vi "SiCM.vi"() -> ()   [LabVIEW 2016]
doc: "SICM module for Hopping Mode.\nRunning this VI takes the control over the PID (ZController). But closing it by clicking on the Cross in the corner of the window releases the PID which is accessible again.\nTo use the motor and the auto-approach module, the window ZController should be used while the SICM Hopping window is running. The Z Controller window will do the Auto-Approach by turning on and off the Hopping movement."
uses:
  controls/Enum.ctl
  <vilib>/rvi/interface/common/niFpgaWaitOnOcc.vi
  <vilib>/rvi/errors/niLvFpgaAdjustHostInterfaceError.vi
  <vilib>/RVI Host/nirviSupport.llb/nirviErrorClusterFromErrorCode.vi
  <vilib>/rvi/interface/nirviMethod/nirviMethod.xnode
  controls/FPGAVIreferenceTypeDef.ctl
  FPGA Bitfiles/qnmController797_usbRIO_controllerFPGAmu.lvbitx
  <vilib>/rvi/interface/nirviReadWriteControl/nirviReadWriteControl.xnode
  <vilib>/regexp/Match Regular Expression.xnode
  controls/FPGAVIreferenceTypeDefScanEngine.ctl
  Course Project/support/Message Queue/Message Queue.lvlib
  <vilib>/rvi/errors/niLvFpgaMergeErrorWithErrorCode.vi
  Course Project/support/User Event - Stop/User Event - Stop.lvlib
  <vilib>/FPGAPlugInAG/USB-7856R OEM/niLvFpga_AcknowledgeIrq_USB-7856R OEM.vi
  NiFpgaLv.dll
  <vilib>/FPGAPlugInAG/USB-7856R OEM/niLvFpga_ReadFifo_USB-7856R OEM.vi
  <vilib>/FPGAPlugInAG/USB-7856R OEM/niLvFpga_ConfigureFifo_USB-7856R OEM.vi
  <vilib>/FPGAPlugInAG/USB-7856R OEM/niLvFpga_StartFifo_USB-7856R OEM.vi
  <vilib>/rvi/interface/nirviMethod/StockFPGA_InlinedMethodWaitForSingleIRQ.vi
  <vilib>/FPGAPlugInAG/USB-7856R OEM/niLvFpga_WaitOnIrq_USB-7856R OEM.vi
  <vilib>/FPGAPlugInAG/USB-7856R OEM/niLvFpga_StopFifo_USB-7856R OEM.vi
panel:
  out "Progress":u8(slide) scale=0.0..100.0
  out "Cursor":dbl format="%#_3pm"
  out "Trig Height":dbl=1.0953788757324218e-07 format="%#_3pm"
  in  "Plots":T1={"Current"=TRUE, "Baseline"=TRUE, "Height"=TRUE, "TrigHeight"=TRUE}
  in  "Real Time":bool
  in  "Update":i32=20 format="%.0fms"
  in  "Window":cluster{"Window":dbl}={"Window"=0.005} {"Window" format="%_3ps"}
  out "Baseline":dbl=0.9660243988037109 format="%#_3p"
  out "Height":dbl=-5.129915237426758e-07 format="%#_3pm"
  out "Current":dbl=0.96649169921875 format="%#_3p"
  in  "SICM":enum32{"Hopping", "IV Curve"}(tab)
  in  "Retract period":dbl=0.002048131080389145 format="%#_3ps"
  in  "Enable?":bool caption="Enable"
  in  "Setpoint":sgl=99.0 min=0 max=100 format="%_3g%"
  in  "Retract height":dbl=2e-06 min=0.0 max=5e-06 format="%_3pm"
  in  "Approach rate":dbl=0.0001 format="%_3pm/s"
  in  "Adaptive":bool=TRUE
  in  "Retract delay":dbl=0.0009379999999999996 min=1e-09 format="%_3ps"
  in  "Adaptive min":dbl=9.0 format="%#_3f%"
  in  "Average period":dbl=0.001 min=1e-09 format="%_3ps"
  in  "Time constant":dbl=3.0 min=1e-09 format="%#_3ps"
  in  "Delta":dbl=5.55e-05 format="%_3p"
  in  "Relative":bool=TRUE
  in  "Ramp":bool caption="Enable"
  out "Inner radius":dbl format="%#_3pm"
  out "Resistance":dbl format="%#_3pOhm"
  out "Z":dbl=0.1 format="%.0pV"
  out "XY":dbl=0.1 format="%.0pV"
  out "R²":dbl=0.1 format="%_3f%"
  in  "IVParameters":T2={"Solution"="140", "Gain"=1.0, "Conductivity"=140.0, "Apex Angle"=5.0, "Points"=100, "Voltage\nRamp"={"Min"=-3.0, "Max"=3.0}} {"Voltage\nRamp"."Min" format="%#_3pV"; "Voltage\nRamp"."Max" format="%#_3pV"; "Points" format="%#.0f"; "Apex Angle" format="%#_3pdeg"; "Conductivity" format="%#_3pS/m"; "Gain" format="%#_3p"}
  out "IV Curve":cluster{dbl[], dbl[]}(graph)
  in  "Reset":bool
  out "Graph":waveform(dbl)[](graph)
  out "RT Graph":dbl[][](graph)
  # "Baseline"
  # "Hopping"
  # "Baseline"
  # "Resolution"
  # "Display"
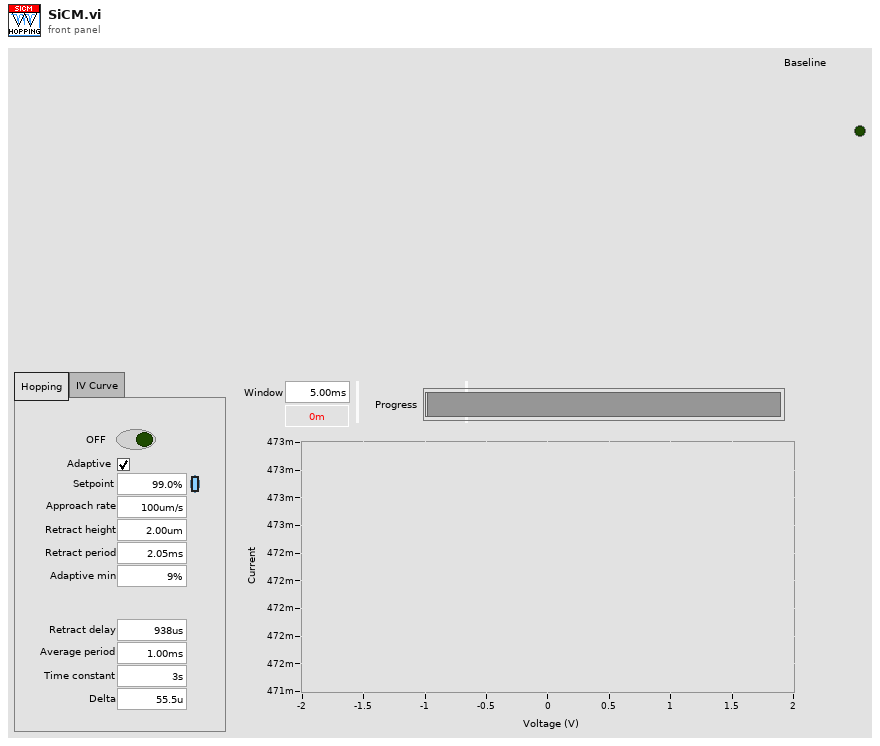
[diagram p1: front panel]
types:
  T1 = cluster{"Current":bool, "Baseline":bool, "Height":bool, "TrigHeight":bool}
  T2 = cluster{"Solution":string, "Gain":dbl, "Conductivity":dbl, "Apex Angle":dbl, "Points":i32, "Voltage\nRamp":cluster{"Min":dbl, "Max":dbl}}
  T3 = typedef "Enum.ctl" = enum16{"Init", "Read", "Write"}
  T4 = cluster{"calibName":string[], "calibParameters":cluster{"Sensitivity":cluster{"Sens X":dbl, "Sens Y":dbl, "Sens Z":dbl}, "Range":cluster{"Range X":dbl, "Range Y":dbl, "Range Z":dbl}, "HV gain":cluster{"HV gain X":dbl, "HV gain Y":dbl, "HV gain Z":dbl}}[], "calibIndex":i32}
  T5 = cluster{"Sensitivity":cluster{"Sens X":dbl, "Sens Y":dbl, "Sens Z":dbl}, "Range":cluster{"Range X":dbl, "Range Y":dbl, "Range Z":dbl}, "HV gain":cluster{"HV gain X":dbl, "HV gain Y":dbl, "HV gain Z":dbl}}[]
  T6 = typedef "FPGAVIreferenceTypeDef.ctl" = refnum<k20>
  T7 = cluster{"Sensitivity":cluster{"Sens X":dbl, "Sens Y":dbl, "Sens Z":dbl}, "Range":cluster{"Range X":dbl, "Range Y":dbl, "Range Z":dbl}, "HV gain":cluster{"HV gain X":dbl, "HV gain Y":dbl, "HV gain Z":dbl}}
  T8 = typedef "Message Queue.lvlib/All Message Queues.ctl" = cluster{"IU":refnum<queue>}
  T9 = typedef "FPGAVIreferenceTypeDefScanEngine.ctl" = refnum<k20>
  T10 = cluster{"write":bool, "data":fxp<+,16,1>, "index":u16}
  T11 = enum8{"Enabled", "Disabled", "Disabled and Grayed Out"}
  T12 = cluster{"inverseDecimation":fxp<+,22,0>, "decimation":u16, "waveSize":u16, "pixelDecimation":u16}
  T13 = cluster{"sicm.p.enable":bool, "sicm.p.adaptiveStepDown":bool, "sicm.p.relSetpoint":bool}
  T14 = cluster{"sicm.p.setPoint":fxp<+,20,0>, "sicm.p.setPointFrac":fxp<+/-,20,14>, "stepDown":fxp<+/-,28,4>, "retractHeight":fxp<+/-,28,4>, "adaptiveMin":fxp<+,10,0>}
  T15 = cluster{"scanEngineHz":u32, "feedbackHz":u32, "sicmHz":u32, "rampHz":u32}
  T16 = cluster{"se.blc.p.postRetractDelay":u16, "se.blc.p.windowSize":u16, "se.blc.p.updateFactor":i16, "blc.resetBackground":bool, "se.blc.p.mindelta":fxp<+/-,12,-14>}
  T17 = cluster{"hdt.int.s.transferSource":u8, "hdt.int.p.useInternalMemStartPos":bool, "hdt.int.p.memStartPos":fxp<+,14,14>, "hdt.int.p.readLength":u16, "hdt.int.p.readFwd":bool, "hdt.int.p.memReadDec":u16, "hdt.int.p.startTransfer":bool}
  T18 = cluster{"sicm.ptsAfterTrig":u16, "sicm.p.memorywWriteDec":u16}
  T19 = cluster{"feedbackHz":u32, "sicm.display.sicm.p.memorywWriteDec":u16}
  T20 = cluster{"carryOut":fxp<+/-,22,2>, "1/x":fxp<+/-,32,24>, "x*y":fxp<+,24,1>}
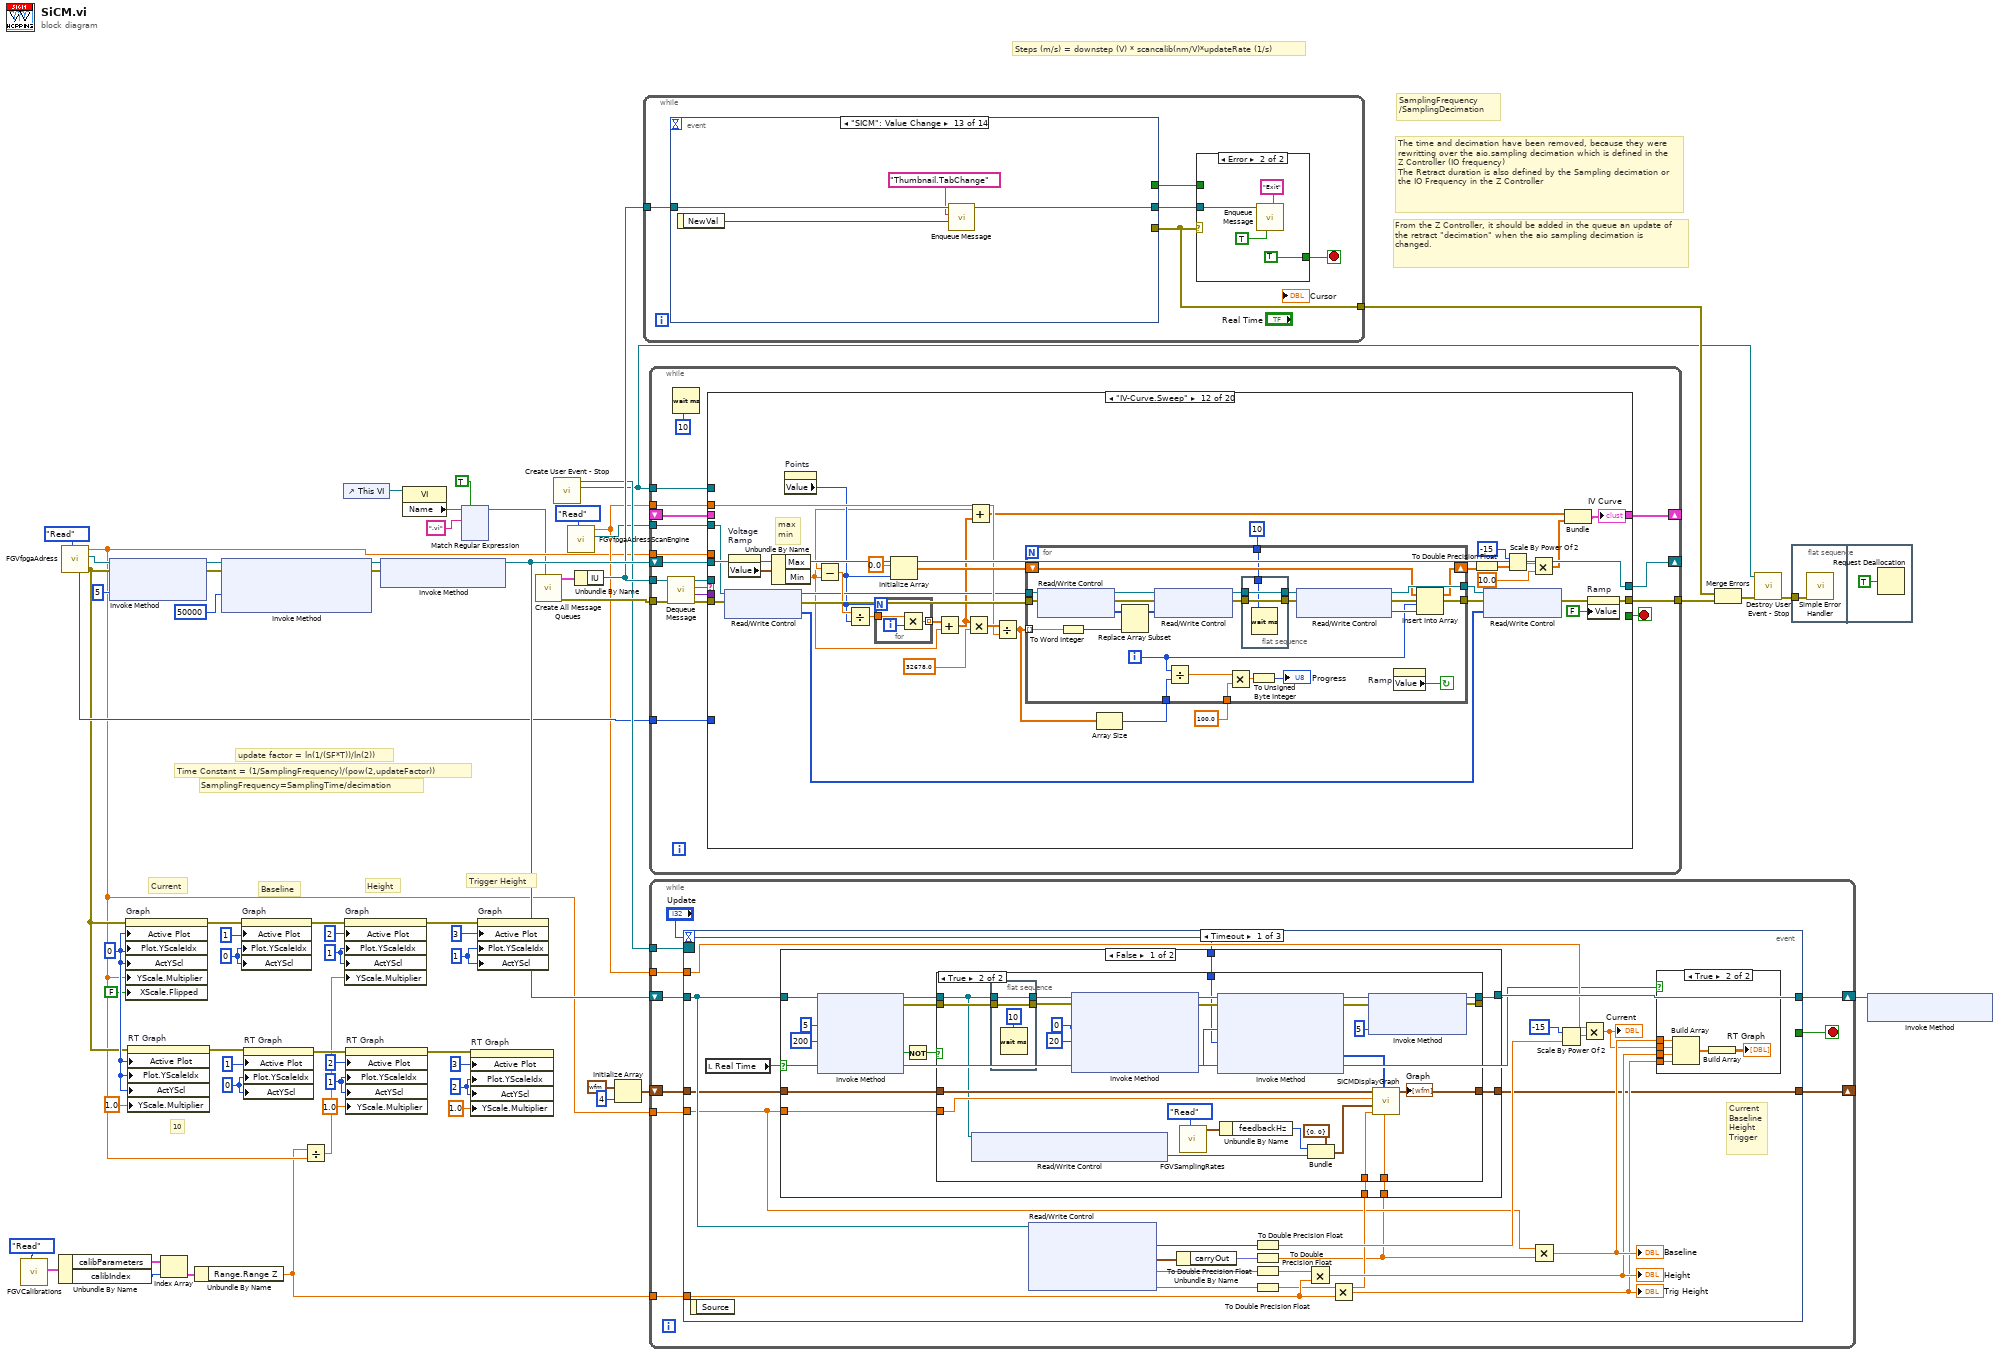
[diagram p0: block diagram]
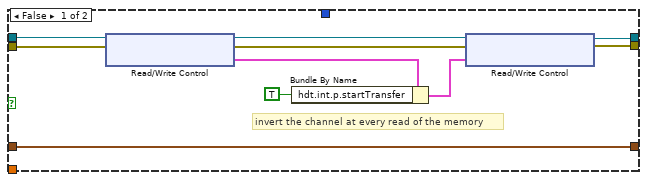
[diagram p2: hidden frame]
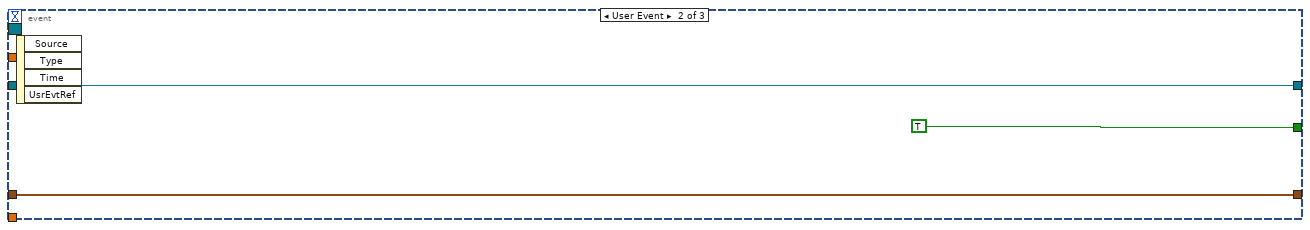
[diagram p5: hidden frame]
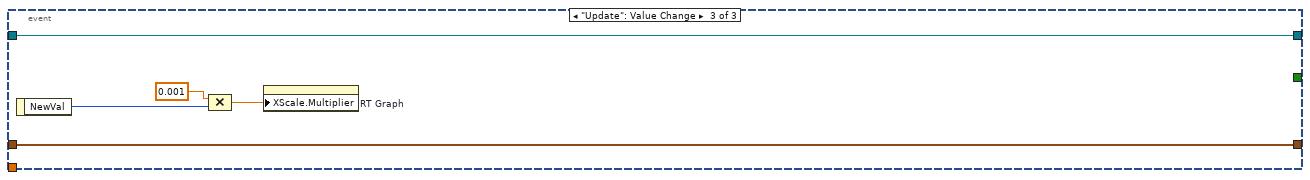
[diagram p6: hidden frame]
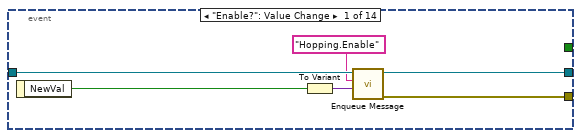
[diagram p8: hidden frame]
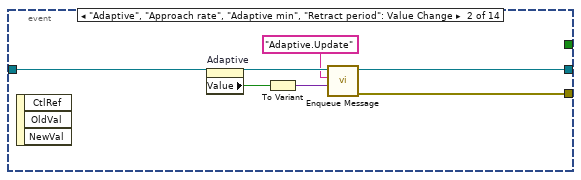
[diagram p9: hidden frame]
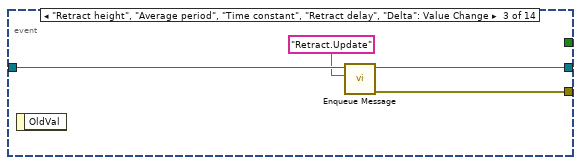
[diagram p10: hidden frame]
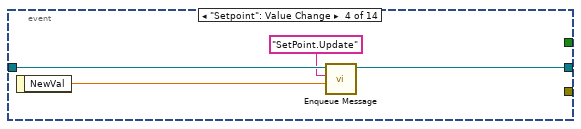
[diagram p11: hidden frame]
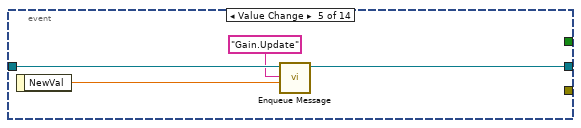
[diagram p12: hidden frame]
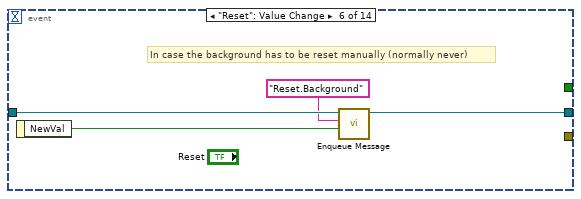
[diagram p13: hidden frame]
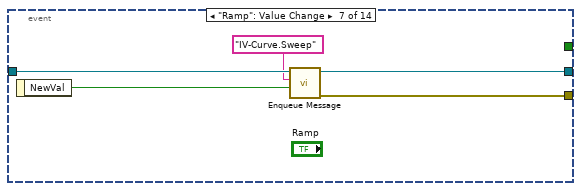
[diagram p14: hidden frame]
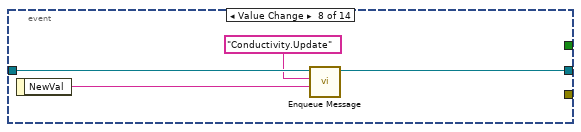
[diagram p15: hidden frame]
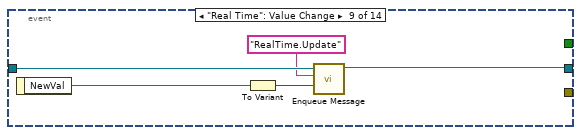
[diagram p16: hidden frame]
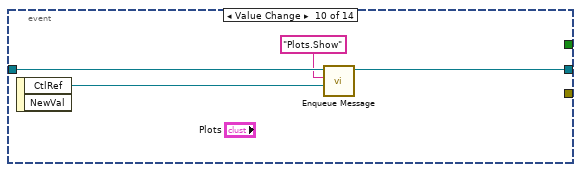
[diagram p17: hidden frame]
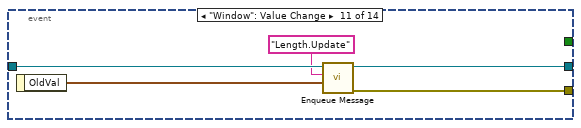
[diagram p18: hidden frame]
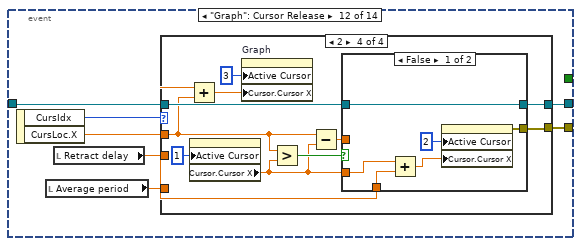
[diagram p19: hidden frame]
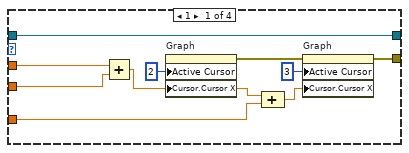
[diagram p20: hidden frame]
diagram:
  w20 = 2 ("Active Y Scale")
  w23 = 1 ("Active Y Scale")
  w26 = 0 ("Active Y Scale")
  w31 = 1 ("Active Y Scale")
  w33 = 1 ("Active Y Scale")
  w27 = u32 0 ("Active Plot")
  w35 = 0 ("Active Y Scale")
  # "10"
  # "Baseline"
  # "Current"
  # "Trigger Height"
  # "Height"
  # "From the Z Controller, it should be added in the queue an update of the retract \"decimation\" when the aio sampling decimation is changed."
  # "The time and decimation have been removed, because they were rewritting over the aio.sampling decimation which is defined in the Z Controller (IO frequency)\nThe Retract duration is also defined by the Sampling decimation or the IO Frequency in the Z Controller"
  # "SamplingFrequency\n/SamplingDecimation"
  # "SamplingFrequency=SamplingTime/decimation"
  # "update factor = ln(1/(SF*T))/ln(2))"
  # "Time Constant = (1/SamplingFrequency)/(pow(2,updateFactor))"
  # "Steps (m/s) = downstep (V) * scancalib(nm/V)*updateRate (1/s)"
  n1 = call "FGVCalibrations.vi"("Enum"=Enum."Read") -> ("calibOut"=w38:T4)  [unwired: 9 in, 1 out]
  n2 = Unbundle By Name(w38) -> ("calibParameters"=w39:T5, "calibIndex"=w41:i32)
  n3 = call "FGVfpgaAdress.vi"("Enum"=Enum."Read") -> ("error out"=w17:errorcluster, "FPGA VI Reference Out"=w61:T6, "voltageRange(+/-)Out"=w14:dbl, "ioFreqHzOut"=w44:u32)  [unwired: 5 in, 2 out]
  n4 = xnode "Invoke Method"("FPGA VI Reference In"=w61, "error in"=w17, "IRQ Number(s)"=5) -> ("FPGA VI Reference Out"=w50:T6, "error out"=w51:errorcluster)
  n5 = property on="Graph" class="WFGraph (strict)"(error in=w17, "Active Plot"=w27, "Plot.YScaleIdx"=w27, "ActYScl"=w27, "YScale.Multiplier"=w14, "XScale.Flipped"=FALSE ("X Scale.Flipped")) -> (error out=w30:errorcluster)  [unwired: 1 in, 1 out]
  n6 = property on="RT Graph" class="WFChart (strict)"(error in=w17, "Active Plot"=w27, "Plot.YScaleIdx"=w27, "ActYScl"=w27, "YScale.Multiplier"=1.0 ("Y Scale.Offset and Multiplier:Multiplier")) -> (error out=w24:errorcluster)  [unwired: 1 in, 1 out]
  n7 = Index Array(array=w39, index=w41) -> (element=w40:T7)
  n8 = Unbundle By Name(w40) -> ("Range.Range Z"=w11:dbl)
  n9 = xnode "Invoke Method"("FPGA VI Reference In"=w50, "error in"=w51, "Requested Depth"=u32 50000) -> ("FPGA VI Reference Out"=w55:T6, "error out"=w53:errorcluster)  [unwired: 1 out]
  n10 = property on="Graph" class="WFGraph (strict)"(error in=w30, "Active Plot"=u32 1, "Plot.YScaleIdx"=w35, "ActYScl"=w35) -> (error out=w29:errorcluster)  [unwired: 1 in, 1 out]
  n11 = property on="RT Graph" class="WFChart (strict)"(error in=w24, "Active Plot"=u32 1, "Plot.YScaleIdx"=w26, "ActYScl"=w26) -> (error out=w21:errorcluster)  [unwired: 1 in, 1 out]
  n12 = Divide(x=w11, y=w14) -> (x/y=w13:dbl)
  n13 = control-ref of="This VI"() -> (w5:refnum<vi>)
  n14 = property on="Graph" class="WFGraph (strict)"(error in=w29, "Active Plot"=u32 2, "Plot.YScaleIdx"=w33, "ActYScl"=w33, "YScale.Multiplier"=w13) -> (error out=w28:errorcluster)  [unwired: 1 in, 1 out]
  n15 = property on="RT Graph" class="WFChart (strict)"(error in=w21, "Active Plot"=u32 2, "Plot.YScaleIdx"=w23, "ActYScl"=w23, "YScale.Multiplier"=1.0 ("Y Scale.Offset and Multiplier:Multiplier")) -> (error out=w18:errorcluster)  [unwired: 1 in, 1 out]
  n16 = xnode "Invoke Method"("FPGA VI Reference In"=w55, "error in"=w53) -> ("FPGA VI Reference Out"=w63:T6)  [unwired: 1 out]
  n17 = property class="VI"(reference=w5) -> ("Name"=w4:string)  [unwired: 1 in, 2 out]
  n18 = xnode "Match Regular Expression"("input string"=w4, "regular expression"=".vi", "ignore case? (F)"=TRUE) -> ("before match"=w2:string)  [unwired: 3 in, 4 out]
  n19 = property on="RT Graph" class="WFChart (strict)"(error in=w18, "Active Plot"=u32 3, "Plot.YScaleIdx"=w20, "ActYScl"=w20, "YScale.Multiplier"=1.0 ("Y Scale.Offset and Multiplier:Multiplier")) -> ()  [unwired: 1 in, 2 out]
  n20 = property on="Graph" class="WFGraph (strict)"(error in=w28, "Active Plot"=u32 3, "Plot.YScaleIdx"=w31, "ActYScl"=w31) -> ()  [unwired: 1 in, 2 out]
  n21 = call "Create All Message Queues.vi"("QueueName"=w2) -> ("ErrorOut"=w58:errorcluster, "MessageQueueOut"=w60:T8)  [unwired: 9 in]
  n22 = call "Create User Event - Stop.vi"() -> ("Événement utilisateur - Arrêt"=w46:refnum<user-event>, "Refnum Enregistrement à l'événement Arrêt"=w49:refnum<event-registration>)  [unwired: 9 in, 1 out]
  n23 = call "FGVfpgaAdressScanEngine.vi"("Enum"=Enum."Read") -> ("FPGA.SEout"=w45:T9, "voltageRange(+/-)Out"=w42:dbl)  [unwired: 6 in, 3 out]
  n24 = Unbundle By Name(w60) -> ("IU"=w59:refnum<queue>)
  n25 = Initialize Array(waveform(dbl) {"t0"=timestamp(0 s since 1904-01-01), "dt"=1.0, "Y"=[0.0]}, 4 ("dimension size")) -> (w8:waveform(dbl)[])
  n26 = while {
    tunnel: w59 -> [w68]
    tunnel: [w64] -> w56
    stop <- w66 stop-if-true
    n27 = event shown="[12] \"SICM\": Value Change" {
      selector: _ -> [_ _ _ _ _ _ _ _ _ _ _ _ _ _]
      dyn-events: _ -> [_ _ _ _ _ _ _ _ _ _ _ _ _ _]
      timeout: _ -> [_ _ _ _ _ _ _ _ _ _ _ _ _ _]
      tunnel: [_ _ _ _ _ _ _ _ _ _ _ _ _ w197] -> w67
      tunnel: w68 -> [w79 w85 w89 w93 w97 w101 w106 w110 w115 w119 w124 w131 w191 w193]
      tunnel: [w76 w82 w86 _ _ _ w103 _ _ _ w121 w127 _ _] -> w64
      tunnel: [w78 w83 w87 w91 w96 w100 w104 w109 w114 w118 w122 w130 w190 w192] -> w65
      event "Enable?": Value Change {
        n28 = event-data() -> ("NewVal"=w75:bool)  [unwired: 1 in]
        n29 = To Variant(anything=w75) -> (Variant=w74:variant)
        n30 = call "Enqueue Message.vi"("Data"=w74, "Message"="Hopping.Enable", "Queue"=w79) -> ("error out"=w76:errorcluster, "Queue dup."=w78:refnum<queue>)  [unwired: 7 in]
      }
      event "Adaptive", "Approach rate", "Adaptive min", "Retract period": Value Change {
        n31 = event-data() -> ()  [unwired: 1 in, 3 out]
        n32 = property on="Adaptive" class="Bool (strict)"() -> ("Value"=w81:bool)  [unwired: 2 in, 2 out]
        n33 = To Variant(anything=w81) -> (Variant=w80:variant)
        n34 = call "Enqueue Message.vi"("Data"=w80, "Message"="Adaptive.Update", "Queue"=w85) -> ("error out"=w82:errorcluster, "Queue dup."=w83:refnum<queue>)  [unwired: 7 in]
      }
      event "Retract height", "Average period", "Time constant", "Retract delay", "Delta": Value Change {
        n35 = event-data() -> ()  [unwired: 1 in, 1 out]
        n36 = call "Enqueue Message.vi"("Message"="Retract.Update", "Queue"=w89) -> ("error out"=w86:errorcluster, "Queue dup."=w87:refnum<queue>)  [unwired: 8 in]
      }
      event "Setpoint": Value Change {
        n37 = event-data() -> ("NewVal"=w90:sgl)  [unwired: 1 in]
        n38 = call "Enqueue Message.vi"("Data"=w90, "Message"="SetPoint.Update", "Queue"=w93) -> ("Queue dup."=w91:refnum<queue>)  [unwired: 7 in, 1 out]
      }
      event "IVParameters.Gain": Value Change {
        n39 = event-data() -> ("NewVal"=w94:dbl)  [unwired: 1 in]
        n40 = call "Enqueue Message.vi"("Data"=w94, "Message"="Gain.Update", "Queue"=w97) -> ("Queue dup."=w96:refnum<queue>)  [unwired: 7 in, 1 out]
      }
      event "Reset": Value Change {
        # "In case the background has to be reset manually (normally never)"
        n41 = event-data() -> ("NewVal"=w98:bool)  [unwired: 1 in]
        n42 = call "Enqueue Message.vi"("Data"=w98, "Message"="Reset.Background", "Queue"=w101) -> ("Queue dup."=w100:refnum<queue>)  [unwired: 7 in, 1 out]
      }
      event "Ramp": Value Change {
        n43 = event-data() -> ("NewVal"=w102:bool)  [unwired: 1 in]
        n44 = call "Enqueue Message.vi"("Data"=w102, "Message"="IV-Curve.Sweep", "Queue"=w106) -> ("error out"=w103:errorcluster, "Queue dup."=w104:refnum<queue>)  [unwired: 7 in]
      }
      event "IVParameters.Solution": Value Change {
        n45 = event-data() -> ("NewVal"=w107:string)  [unwired: 1 in]
        n46 = call "Enqueue Message.vi"("Data"=w107, "Message"="Conductivity.Update", "Queue"=w110) -> ("Queue dup."=w109:refnum<queue>)  [unwired: 7 in, 1 out]
      }
      event "Real Time": Value Change {
        n47 = event-data() -> ("NewVal"=w112:bool)  [unwired: 1 in]
        n48 = To Variant(anything=w112) -> (Variant=w111:variant)
        n49 = call "Enqueue Message.vi"("Data"=w111, "Message"="RealTime.Update", "Queue"=w115) -> ("Queue dup."=w114:refnum<queue>)  [unwired: 7 in, 1 out]
      }
      event "Plots.Current", "Plots.Baseline", "Plots.Height", "Plots.TrigHeight": Value Change {
        n50 = event-data() -> ("CtlRef"=w116:refnum<vi>)  [unwired: 1 in, 1 out]
        n51 = call "Enqueue Message.vi"("Data"=w116, "Message"="Plots.Show", "Queue"=w119) -> ("Queue dup."=w118:refnum<queue>)  [unwired: 7 in, 1 out]
      }
      event "Window": Value Change {
        n52 = event-data() -> ("OldVal"=w120:cluster{"Window":dbl})  [unwired: 1 in]
        n53 = call "Enqueue Message.vi"("Data"=w120, "Message"="Length.Update", "Queue"=w124) -> ("error out"=w121:errorcluster, "Queue dup."=w122:refnum<queue>)  [unwired: 7 in]
      }
      event "Graph": Cursor Release {
        n54 = event-data() -> ("CursIdx"=w129:i32, "CursLoc.X"=w128:dbl)  [unwired: 1 in]
        n55 = local read "Average period"() -> (w125:dbl)
        n56 = local read "Retract delay"() -> (w126:dbl)
        n57 = case shown="2" w129 {
          tunnel: w131 -> [w139 w142 w150 w174]
          tunnel: [w139 w142 w149 w173] -> w130
          tunnel: w128 -> [w140 _ w146 w166]
          tunnel: [w136 _ w148 w172] -> w127
          tunnel: w126 -> [w133 _ _ w164]
          tunnel: w125 -> [w132 _ w143 w165]
          frame 1 {
            n58 = Add(x=w140, y=w133) -> (x+y=w134:dbl)
            n59 = property on="Graph" class="WFGraph (strict)"("Active Cursor"=u32 2, "Cursor.Cursor X"=w134) -> (error out=w137:errorcluster)  [unwired: 2 in, 1 out]
            n60 = Compound Arithmetic op=ADD(w134, w132) -> (w135:dbl)
            n61 = property on="Graph" class="WFGraph (strict)"(error in=w137, "Active Cursor"=u32 3, "Cursor.Cursor X"=w135) -> (error out=w136:errorcluster)  [unwired: 1 in, 1 out]
          }
          frame 0, Default {
          }
          frame 3 {
            n62 = property on="Graph" class="WFGraph (strict)"("Active Cursor"=u32 2) -> ("Cursor.Cursor X"=w144:dbl)  [unwired: 2 in, 2 out]
            n63 = Greater?(x=w146, y=w144) -> (0:w151:bool)
            n64 = Subtract(x=w146, y=w144) -> (x-y=w145:dbl)
            n65 = case shown="False" w151 {
              tunnel: w150 -> [w157 w163]
              tunnel: [w157 w162] -> w149
              tunnel: [w155 w161] -> w148
              tunnel: w145 -> [_ w158]
              tunnel: w144 -> [w152 _]
              tunnel: w143 -> [w153 _]
              frame False {
                n66 = Add(x=w152, y=w153) -> (x+y=w154:dbl)
                n67 = property on="Graph" class="WFGraph (strict)"("Active Cursor"=u32 4, "Cursor.Cursor X"=w154) -> (error out=w155:errorcluster)  [unwired: 2 in, 1 out]
              }
              frame True {
                n68 = property on="Average period" class="DigNum (strict)"("Value"=w158) -> (error out=w159:errorcluster)  [unwired: 2 in, 1 out]
                n69 = call "Enqueue Message.vi"("error in"=w159, "Message"="Retract.Update", "Queue"=w163) -> ("error out"=w161:errorcluster, "Queue dup."=w162:refnum<queue>)  [unwired: 7 in]
              }
            }
          }
          frame 2 {
            n70 = Add(x=w165, y=w166) -> (x+y=w167:dbl)
            n71 = property on="Graph" class="WFGraph (strict)"("Active Cursor"=u32 1) -> ("Cursor.Cursor X"=w169:dbl)  [unwired: 2 in, 2 out]
            n72 = property on="Graph" class="WFGraph (strict)"("Active Cursor"=u32 3, "Cursor.Cursor X"=w167) -> ()  [unwired: 2 in, 2 out]
            n73 = Greater?(x=w166, y=w169) -> (0:w175:bool)
            n74 = Subtract(x=w166, y=w169) -> (x-y=w170:dbl)
            n75 = case shown="False" w175 {
              tunnel: w174 -> [w181 w187]
              tunnel: [w181 w186] -> w173
              tunnel: [w179 w185] -> w172
              tunnel: w170 -> [_ w182]
              tunnel: w169 -> [w176 _]
              tunnel: w164 -> [w177 _]
              frame False {
                n76 = Add(x=w176, y=w177) -> (x+y=w178:dbl)
                n77 = property on="Graph" class="WFGraph (strict)"("Active Cursor"=u32 2, "Cursor.Cursor X"=w178) -> (error out=w179:errorcluster)  [unwired: 2 in, 1 out]
              }
              frame True {
                n78 = property on="Retract delay" class="DigNum (strict)"("Value"=w182) -> (error out=w183:errorcluster)  [unwired: 2 in, 1 out]
                n79 = call "Enqueue Message.vi"("error in"=w183, "Message"="Retract.Update", "Queue"=w187) -> ("error out"=w185:errorcluster, "Queue dup."=w186:refnum<queue>)  [unwired: 7 in]
              }
            }
          }
        }
      }
      event "SICM": Value Change {
        n80 = event-data() -> ("NewVal"=w188:enum32{"Hopping", "IV Curve"})  [unwired: 1 in]
        n81 = call "Enqueue Message.vi"("Data"=w188, "Message"="Thumbnail.TabChange", "Queue"=w191) -> ("Queue dup."=w190:refnum<queue>)  [unwired: 7 in, 1 out]
      }
      event Panel Close? {
        w197 = TRUE ("Rejeter ?")
        n82 = event-data() -> ()  [unwired: 1 in, 1 out]
        n83 = Flush Queue(queue=w193) -> (queue out=w199:refnum<queue>)  [unwired: 1 in, 2 out]
        n84 = call "Enqueue Message.vi"("Data"=FALSE, "Message"="Hopping.Enable", "Queue"=w199) -> ("Queue dup."=w198:refnum<queue>)  [unwired: 7 in, 1 out]
        n85 = call "Enqueue Message.vi"("Message"="Exit", "Queue"=w198) -> ("Queue dup."=w192:refnum<queue>)  [unwired: 8 in, 1 out]
        n86 = event-data ("Event Filter Node")("Discard?"=w197) -> ()  [unwired: 1 in, 1 out]
      }
    }
    n87 = case shown="Error" w64 {
      tunnel: [w69 TRUE ("Rejeter ?")] -> w66
      tunnel: w67 -> [w69 _]
      tunnel: w65 -> [_ w72]
      frame No Error {
      }
      frame Error {
        n88 = call "Enqueue Message.vi"("Prioritary message"=TRUE ("Message prioritaire ? (F)"), "Message"="Exit", "Queue"=w72) -> ()  [unwired: 7 in, 2 out]
      }
    }
  }
  n89 = while {
    tunnel: w59 -> [w211]
    tunnel: w58 -> [w215]
    tunnel: [w216] -> w57
    shift-right: [w208] -> _
    shift-left: w63 -> [w209]
    tunnel: w44 -> [w207]
    tunnel: w46 -> [w205]
    tunnel: w45 -> [w204]
    tunnel: w42 -> [w203]
    tunnel: w14 -> [w206]
    shift-right: [w202] -> _
    shift-left: _ -> [w201]
    stop <- w217 stop-if-true
    n90 = call "Dequeue Message.vi"("entrée d'erreur (pas d'erreur)"=w215, "File d'attente de messages"=w211) -> ("sortie d'erreur"=w214:errorcluster, "Données de message"=w213:variant, "Message"=w210:string, "File d'attente de message dup."=w212:refnum<queue>)  [unwired: 6 in]
    n91 = Wait (ms)(milliseconds to wait=u32 10) -> ()  [unwired: 1 out]
    n92 = case "Conditions des messages" shown="\"IV-Curve.Sweep\"" w210 {
      selector: w210 -> [_ _ _ _ _ _ _ _ _ _ _ _ _ _ _ _ _ _ _ w748]
      tunnel: w212 -> [_ w261 _ _ _ _ _ _ _ _ _ _ _ _ _ _ _ w726 w742 _]
      tunnel: w214 -> [w220 w240 w283 w329 w379 w424 w441 w459 w493 w510 w518 w533 w609 w635 w653 w673 w697 w718 w741 _]
      tunnel: [w220 w222 w273 w332 w371 w426 w446 w455 w498 w512 w518 w536 w599 w630 w647 w666 w687 w716 w732 w746] -> w216
      tunnel: [_ _ _ _ _ _ _ _ _ _ _ _ _ _ _ _ _ _ TRUE _] -> w217
      tunnel: w213 -> [_ _ _ w331 w354 _ w438 w457 w476 _ _ _ _ w634 w652 w670 w695 _ _ _]
      tunnel: w209 -> [w219 w259 w282 w320 w370 w425 w447 w460 w503 w511 w517 w554 w608 w636 w655 w672 w702 w723 w739 w744]
      tunnel: [w219 w259 w274 w323 w372 w427 w445 w460 w499 w513 w517 w554 w600 w636 w655 w672 w702 w723 w738 w744] -> w208
      tunnel: w207 -> [_ _ _ _ _ _ _ _ _ _ _ _ _ _ _ _ _ _ _ _]
      tunnel: w206 -> [_ _ _ _ w338 _ _ _ _ _ _ _ _ _ _ _ _ _ _ _]
      tunnel: w205 -> [_ _ _ _ _ _ _ _ _ _ _ _ _ _ _ _ _ _ w735 _]
      tunnel: w204 -> [_ _ _ _ _ _ _ _ _ _ _ w532 _ _ _ _ _ _ _ _]
      tunnel: w203 -> [_ _ _ _ _ _ _ _ _ _ _ w538 w588 _ _ _ _ _ _ _]
      tunnel: [w218 w265 w279 w321 w351 w407 w436 w453 w494 w506 w516 w537 w604 w629 w654 w671 w701 w722 w729 w743] -> w202
      tunnel: w201 -> [w218 w265 w279 w321 w351 w407 w436 w453 w494 w506 w516 _ w604 w629 w654 w671 w701 w722 w729 w743]
      frame "--------- Initialization ---------" {
      }
      frame "Initialize" {
        n93 = call "Enqueue Message.vi"("error in"=w240, "Message"="RealTime.Update", "Queue"=w261) -> ("error out"=w238:errorcluster, "Queue dup."=w262:refnum<queue>)  [unwired: 7 in]
        n94 = To Variant(anything="SICM") -> (Variant=w232:variant)
        n95 = local write "Enable?"(FALSE ("Enable?")) -> ()
        n96 = call "Enqueue Message.vi"("error in"=w238, "Data"=w232, "Message"="Thumbnail.TabChange", "Queue"=w262) -> ("error out"=w267:errorcluster, "Queue dup."=w266:refnum<queue>)  [unwired: 6 in]
        n97 = call "Enqueue Message.vi"("error in"=w267, "Data"=TRUE, "Message"="Hopping.Enable", "Queue"=w266) -> ("error out"=w263:errorcluster, "Queue dup."=w264:refnum<queue>)  [unwired: 6 in]
        n98 = call "Enqueue Message.vi"("error in"=w263, "Data"=FALSE, "Message"="Hopping.Enable", "Queue"=w264) -> ("error out"=w223:errorcluster, "Queue dup."=w268:refnum<queue>)  [unwired: 6 in]
        n99 = call "Enqueue Message.vi"("error in"=w223, "Message"="FPGA.Initialize", "Queue"=w268) -> ("error out"=w269:errorcluster, "Queue dup."=w270:refnum<queue>)  [unwired: 7 in]
        n100 = To Variant(anything="Window") -> (Variant=w226:variant)
        n101 = call "Enqueue Message.vi"("error in"=w269, "Data"=w226, "Message"="Length.Update", "Queue"=w270) -> ("error out"=w221:errorcluster, "Queue dup."=w271:refnum<queue>)  [unwired: 6 in]
        n102 = call "Enqueue Message.vi"("error in"=w221, "Data"=TRUE, "Message"="Adaptive.Update", "Queue"=w271) -> ("error out"=w249:errorcluster, "Queue dup."=w257:refnum<queue>)  [unwired: 6 in]
        n103 = call "Enqueue Message.vi"("error in"=w249, "Message"="Retract.Update", "Queue"=w257) -> ("error out"=w248:errorcluster, "Queue dup."=w256:refnum<queue>)  [unwired: 7 in]
        n104 = To Variant(anything="Setpoint") -> (Variant=w234:variant)
        n105 = call "Enqueue Message.vi"("error in"=w248, "Data"=w234, "Message"="SetPoint.Update", "Queue"=w256) -> ("error out"=w247:errorcluster, "Queue dup."=w255:refnum<queue>)  [unwired: 6 in]
        n106 = call "Enqueue Message.vi"("error in"=w247, "Message"="Bias.Update", "Queue"=w255) -> ("error out"=w245:errorcluster, "Queue dup."=w258:refnum<queue>)  [unwired: 7 in]
        n107 = call "Enqueue Message.vi"("error in"=w245, "Message"="Time.Update", "Queue"=w258) -> ("error out"=w231:errorcluster, "Queue dup."=w260:refnum<queue>)  [unwired: 7 in]
        n108 = property on="Solution" class="CmbBox"() -> ("Value"=w230:string)  [unwired: 2 in, 2 out]
        n109 = To Variant(anything=w230) -> (Variant=w229:variant)
        n110 = call "Enqueue Message.vi"("error in"=w231, "Data"=w229, "Message"="Conductivity.Update", "Queue"=w260) -> ("error out"=w222:errorcluster)  [unwired: 6 in, 1 out]
      }
      frame "FPGA.Initialize" {
        w272 = u8 1 items=["process Variable", "SICM", "ramp"] ("flt.i.bypassSource")
        w292 = u16 128 ("numRoundingPts")
        w276 = u8 1 items=["PID/ORT", "SICM"] ("hdt.mainOutStreamSelect")
        n111 = for {
          N: 4 -> [_]
          shift-right: [w312] -> _
          shift-left: u32 0 ("Elements Remaining") -> [w313]
          tunnel: [w310] -> w280
          tunnel: 20 ("Timeout (ms)") -> [w311]
          tunnel: [w314] -> w299
          tunnel: w283 -> [w309]
          tunnel: w282 -> [w308]
          n112 = xnode "Invoke Method"("FPGA VI Reference In"=w308, "error in"=w309, "Number of Elements"=w313, "Timeout (ms)"=w311) -> ("FPGA VI Reference Out"=w310:T6, "error out"=w314:errorcluster, "Elements Remaining"=w312:u32)  [unwired: 1 out]
        }
        n113 = To Double Precision Float(number=u16 1 ("numRoundingPts")) -> (double precision float=w288:dbl)
        n114 = call "bangBangMove.vi"("numRoundingPts"=u16 8, "numPts"=w292) -> ("roundedHalfTriangle"=w289:dbl[])  [unwired: 9 in]
        n115 = Build Array (concatenate)(w289, w288) -> (w287:dbl[])
        n116 = for {
          tunnel: w287 -> [w304] mode=indexing
          tunnel: [w303] -> w285
          tunnel: [w302] -> w284
          tunnel: w280 -> [w301]
          tunnel: w299 -> [w300]
          i -> [w305]
          n117 = Bundle By Name(cluster=T10 {"write"=TRUE, "data"=0.0, "index"=0} ("fb.mot.m.motion"), "data"=w304, "index"=w305) -> (w306:T10)
          n118 = xnode "Read/Write Control"("FPGA VI Reference In"=w301, "error in"=w300, "sicm.m.upMotion"=w306) -> ("FPGA VI Reference Out"=w303:T6, "error out"=w302:errorcluster)
        }
        n119 = xnode "Read/Write Control"("FPGA VI Reference In"=w285, "error in"=w284, "sicm.m.upMotion"=T10 {"write"=FALSE, "data"=0.0, "index"=0} ("fb.mot.m.motion"), "fb.p.enable"=FALSE) -> ("FPGA VI Reference Out"=w295:T6, "error out"=w294:errorcluster, "sicm.p.clocks"=w281:T12)
        n120 = Bundle By Name(cluster=w281, "waveSize"=w292) -> (w293:T12)
        n121 = xnode "Read/Write Control"("FPGA VI Reference In"=w295, "error in"=w294, "sicm.p.clocks"=w293, "flt.bypassPI"=FALSE, "flt.i.bypassSource"=w272, "hdt.mainOutStreamSelect"=w276, "hdt.int.p.memWriteSource"=w276, "flt.bypassPI"=TRUE) -> ("FPGA VI Reference Out"=w274:T6, "error out"=w273:errorcluster)
      }
      frame "Hopping.Enable" {
        w315 = u8 1  # SICM
        n122 = Variant To Data(error in=w329, type=TRUE, Variant=w331) -> (data=w322:bool, error out=w318:errorcluster)
        n123 = xnode "Read/Write Control"("FPGA VI Reference In"=w320, "error in"=w318, "flt.i.bypassSource"=w315, "flt.bypassPI"=TRUE) -> ("FPGA VI Reference Out"=w319:T6, "error out"=w317:errorcluster)
        n124 = xnode "Read/Write Control"("FPGA VI Reference In"=w319, "error in"=w317) -> ("FPGA VI Reference Out"=w325:T6, "error out"=w326:errorcluster, "sicm.p.modes"=w328:T13)
        n125 = Bundle By Name(cluster=w328, "sicm.p.enable"=w322) -> (w327:T13)
        n126 = xnode "Read/Write Control"("FPGA VI Reference In"=w325, "error in"=w326, "sicm.p.modes"=w327) -> ("FPGA VI Reference Out"=w323:T6, "error out"=w324:errorcluster)
        n127 = property on="Enable?" class="Bool (strict)"(error in=w324, "Value"=w322) -> (error out=w332:errorcluster)  [unwired: 1 in, 1 out]
      }
      frame "Adaptive.Update" {
        w348 = 100.0  # %
        # "dec = Dt_up*Fio/nPts(waveSize)"
        n128 = Variant To Data(error in=w379, type=TRUE, Variant=w354) -> (data=w333:bool, error out=w355:errorcluster)
        n129 = call "FGVCalibrations.vi"("Enum"=Enum."Read") -> ("calibOut"=w366:T4)  [unwired: 9 in, 1 out]
        n130 = Unbundle By Name(w366) -> ("calibParameters"=w367:T5, "calibIndex"=w369:i32)
        n131 = xnode "Read/Write Control"("FPGA VI Reference In"=w370, "error in"=w355) -> ("FPGA VI Reference Out"=w375:T6, "error out"=w376:errorcluster, "sicm.p.modes"=w373:T13, "sicm.p.params"=w377:T14, "sicm.p.clocks"=w352:T12)
        n132 = call "FGVSamplingRates.vi"("Enum"=Enum."Read") -> ("samplingRatesOut"=w346:T15)  [unwired: 9 in, 1 out]
        n133 = Unbundle By Name(w346) -> ("feedbackHz"=w341:u32)
        n134 = Index Array(array=w367, index=w369) -> (element=w368:T7)
        n135 = Unbundle By Name(w368) -> ("Range.Range Z"=w361:dbl)
        n136 = Unbundle By Name(w352) -> ("waveSize"=w345:u16)
        n137 = Divide(x=w361, y=w338) -> (x/y=w357:dbl)
        n138 = Divide(x=w341, y=w345) -> (x/y=w340:dbl)
        n139 = Multiply(x=w341, y=w357) -> (x*y=w360:dbl)
        n140 = To Unsigned Long Integer(number=w340) -> (unsigned 32bit integer=w334:u32)
        n141 = Reciprocal(x="Retract period") -> (1/x=w339:dbl)
        n142 = call "corerceFPGAClock.vi"("baseClock"=w334, "requestedFrequency"=w339) -> ("decimation"=w380:u16, "realFrequency"=w343:dbl)  [unwired: 7 in, 1 out]
        n143 = Reciprocal(x=w343) -> (1/x=w342:dbl)
        n144 = property on="Retract period" class="DigNum (strict)"("Value"=w342) -> ()  [unwired: 2 in, 2 out]
        n145 = Divide(x="Approach rate", y=w360) -> (x/y=w358:dbl)
        n146 = Bundle By Name(cluster=w373, "sicm.p.adaptiveStepDown"=w333) -> (w374:T13)
        n147 = Select(t=T11."Enabled" ("Disabled"), s=w333, f=T11."Disabled and Grayed Out" ("Disabled")) -> (s? t:f=w335:T11)
        n148 = Divide(x="Adaptive min", y=w348) -> (x/y=w350:dbl)
        n149 = To Fixed-Point(fixed-point type=fxp<+/-,28,4> 0.0 ("stepDown"), number=w358) -> (fixed-point=w356:fxp<+/-,28,4>)
        n150 = property on="Adaptive min" class="DigNum (strict)"("DisabledEnum"=w335) -> ()  [unwired: 2 in, 2 out]
        n151 = Reciprocal(x=w380) -> (1/x=w363:dbl)
        n152 = Bundle By Name(cluster=w377, "stepDown"=w356, "adaptiveMin"=w350) -> (w378:T14)
        n153 = Bundle By Name(cluster=w352, "inverseDecimation"=w363, "decimation"=w380) -> (w362:T12)
        n154 = xnode "Read/Write Control"("FPGA VI Reference In"=w375, "error in"=w376, "sicm.p.modes"=w374, "sicm.p.params"=w378, "sicm.p.clocks"=w362) -> ("FPGA VI Reference Out"=w372:T6, "error out"=w371:errorcluster)
      }
      frame "Retract.Update" {
        # "SamplingFrequency\n/SamplingDecimation"
        n155 = call "FGVCalibrations.vi"("Enum"=Enum."Read") -> ("calibOut"=w412:T4)  [unwired: 9 in, 1 out]
        n156 = call "FGVSamplingRates.vi"("Enum"=Enum."Read") -> ("samplingRatesOut"=w404:T15)  [unwired: 9 in, 1 out]
        n157 = xnode "Read/Write Control"("FPGA VI Reference In"=w425, "error in"=w424) -> ("FPGA VI Reference Out"=w423:T6, "error out"=w430:errorcluster, "sicm.p.params"=w428:T14, "sicm.blc.p.params"=w418:T16)
        n158 = Unbundle By Name(w412) -> ("calibParameters"=w413:T5, "calibIndex"=w415:i32)
        n159 = Unbundle By Name(w404) -> ("feedbackHz"=w403:u32)
        n160 = To Double Precision Float(number=w403) -> (double precision float=w393:dbl)
        n161 = Index Array(array=w413, index=w415) -> (element=w414:T7)
        n162 = Unbundle By Name(w414) -> ("Range.Range Z"=w408:dbl)
        n163 = Multiply(x=2.0, y="Retract height") -> (x*y=w382:dbl)
        n164 = Compound Arithmetic op=MULTIPLY("Retract delay", w393) -> (w420:dbl)
        n165 = Compound Arithmetic op=MULTIPLY("Average period", w393) -> (w421:dbl)
        n166 = Compound Arithmetic op=MULTIPLY(w393, "Time constant") -> (w422:dbl)
        n167 = To Fixed-Point(fixed-point type=fxp<+/-,22,2> 0.0 ("se.blc.p.mindelta"), number="Delta") -> (fixed-point=w387:fxp<+/-,22,2>)
        n168 = expression code="ln(1/x)/ln(2)"(w422) -> (w389:dbl)
        n169 = To Unsigned Word Integer(number=w420) -> (unsigned 16bit integer=w391:u16)
        n170 = To Unsigned Word Integer(number=w421) -> (unsigned 16bit integer=w390:u16)
        n171 = Divide(x=w382, y=w408) -> (x/y=w411:dbl)
        n172 = property on="Retract height" class="DigNum (strict)"("Maximum"=w408, "OutOfRngActMax"=u8 1 ("Response to Value Outside Limits:Maximum")) -> ()  [unwired: 2 in, 2 out]
        n173 = Negate(x=w411) -> (-x=w385:dbl)
        n174 = To Word Integer(number=w389) -> (16bit integer=w388:i16)
        n175 = To Fixed-Point(fixed-point type=fxp<+/-,28,4> 0.0 ("retractHeight"), number=w385) -> (fixed-point=w383:fxp<+/-,28,4>)
        n176 = Bundle By Name(cluster=w418, "se.blc.p.postRetractDelay"=w391, "se.blc.p.windowSize"=w390, "se.blc.p.updateFactor"=w388, "se.blc.p.mindelta"=w387) -> (w417:T16)
        n177 = Bundle By Name(cluster=w428, "retractHeight"=w383) -> (w429:T14)
        n178 = xnode "Read/Write Control"("FPGA VI Reference In"=w423, "error in"=w430, "sicm.p.params"=w429, "sicm.blc.p.params"=w417) -> ("FPGA VI Reference Out"=w427:T6, "error out"=w426:errorcluster)
        n179 = property on="Graph" class="WFGraph (strict)"("Active Cursor"=u32 1) -> ("Cursor.Cursor X"=w397:dbl)  [unwired: 2 in, 2 out]
        n180 = property on="Graph" class="WFGraph (strict)"("Active Cursor"=u32 2) -> ("Cursor.Cursor X"=w400:dbl)  [unwired: 2 in, 2 out]
        n181 = Compound Arithmetic op=ADD(w397, "Retract delay") -> (w398:dbl)
        n182 = Compound Arithmetic op=ADD(w400, "Average period") -> (w399:dbl)
        n183 = property on="Graph" class="WFGraph (strict)"("Active Cursor"=u32 2, "Cursor.Cursor X"=w398) -> ()  [unwired: 2 in, 2 out]
        n184 = property on="Graph" class="WFGraph (strict)"("Active Cursor"=u32 3, "Cursor.Cursor X"=w399) -> ()  [unwired: 2 in, 2 out]
      }
      frame "SetPoint.Update" {
        n185 = Variant To Data(error in=w441, type=sgl 0.0 ("NewVal"), Variant=w438) -> (data=w437:sgl, error out=w440:errorcluster)
        n186 = xnode "Read/Write Control"("FPGA VI Reference In"=w447, "error in"=w440) -> ("FPGA VI Reference Out"=w450:T6, "sicm.p.modes"=w448:T13, "sicm.p.params"=w452:T14)  [unwired: 1 out]
        n187 = Divide(x=w437, y=sgl 100.0) -> (x/y=w434:sgl)
        n188 = expression code="1/(x-1)"(w434) -> (w433:sgl)
        n189 = To Fixed-Point(fixed-point type=fxp<+,20,0> 0.0 ("sicm.p.setPoint"), number=w434) -> (fixed-point=w442:fxp<+,20,0>)
        n190 = To Fixed-Point(fixed-point type=fxp<+/-,20,14> 0.0 ("sicm.p.setPointFrac"), number=w433) -> (fixed-point=w431:fxp<+/-,20,14>)
        n191 = Bundle By Name(cluster=w448, "sicm.p.relSetpoint"=TRUE) -> (w449:T13)
        n192 = Bundle By Name(cluster=w452, "sicm.p.setPoint"=w442, "sicm.p.setPointFrac"=w431) -> (w451:T14)
        n193 = xnode "Read/Write Control"("FPGA VI Reference In"=w450, "sicm.p.modes"=w449, "sicm.p.params"=w451) -> ("FPGA VI Reference Out"=w445:T6, "error out"=w446:errorcluster)  [unwired: 1 in]
      }
      frame "Gain.Update" {
        n194 = Variant To Data(error in=w459, type=0.0 ("NewVal"), Variant=w457) -> (data=w454:dbl, error out=w456:errorcluster)
        n195 = property on="Graph" class="WFGraph (strict)"(error in=w456, "YScale.Multiplier"=w454) -> (error out=w455:errorcluster)  [unwired: 1 in, 1 out]
      }
      frame "Length.Update" {
        w477 = 16000.0  # Maximum length (FPGA)
        w492 = u8 5 items=["memoryChan1", "memoryChan2", "processVarFixedNoPts", "processVarStream", "systemId", "interleaveMemCh1Ch2"] ("hdt.int.s.transferSource")
        n196 = Variant To Data(error in=w493, type=cluster{"Window":dbl} {"Window"=0.0} ("Window"), Variant=w476) -> (data=w474:cluster{"Window":dbl}, error out=w505:errorcluster)
        n197 = call "FGVSamplingRates.vi"("Enum"=Enum."Read") -> ("samplingRatesOut"=w489:T15)  [unwired: 9 in, 1 out]
        n198 = Unbundle By Name(w474) -> ("Window"=w471:dbl)
        n199 = Unbundle By Name(w489) -> ("feedbackHz"=w483:u32)
        n200 = To Double Precision Float(number=w483) -> (double precision float=w466:dbl)
        n201 = xnode "Read/Write Control"("FPGA VI Reference In"=w503, "error in"=w505) -> ("FPGA VI Reference Out"=w500:T6, "hdt.int.p.readParams"=w502:T17, "sicm.display"=w496:T18)  [unwired: 1 out]
        n202 = Multiply(x=w471, y=w466) -> (x*y=w470:dbl)
        n203 = Quotient & Remainder(x=w470, y=w477) -> (floor(x/y)=w462:dbl)  [unwired: 1 out]
        n204 = In Range and Coerce(upper limit=w477, x=w470, lower limit=1.0) -> (coerced(x)=w467:dbl, In Range?=w463:bool)
        n205 = Select(t=1.0, s=w463, f=w462) -> (s? t:f=w461:dbl)
        n206 = Quotient & Remainder(x=w467, y=2.0) -> (floor(x/y)=w469:dbl)  [unwired: 1 out]
        n207 = Reciprocal(x=w466) -> (1/x=w473:dbl)
        n208 = To Unsigned Word Integer(number=w467) -> (unsigned 16bit integer=w482:u16)
        n209 = Multiply(x=w469, y=w461) -> (x*y=w468:dbl)
        n210 = To Unsigned Long Integer(number=w469) -> (unsigned 32bit integer=w472:u32)
        n211 = Multiply(x=w468, y=w473) -> (x*y=w481:dbl)
        n212 = Bundle By Name(cluster=w502, "hdt.int.s.transferSource"=w492, "hdt.int.p.useInternalMemStartPos"=TRUE, "hdt.int.p.readLength"=w482, "hdt.int.p.readFwd"=FALSE, "hdt.int.p.memReadDec"=u16 200) -> (w501:T17)
        n213 = Bundle By Name(cluster=w496, "sicm.ptsAfterTrig"=w472, "sicm.p.memorywWriteDec"=w461) -> (w495:T18)
        n214 = local read "Average period"() -> (w478:dbl)
        n215 = property on="Graph" class="WFGraph (strict)"("Active Cursor"=u32 1, "Cursor.Cursor X"=w481) -> ()  [unwired: 2 in, 2 out]
        n216 = Add(x=w481, y=w478) -> (x+y=w486:dbl)
        n217 = local read "Retract delay"() -> (w479:dbl)
        n218 = property on="Graph" class="WFGraph (strict)"("Active Cursor"=u32 2, "Cursor.Cursor X"=w486) -> ()  [unwired: 2 in, 2 out]
        n219 = xnode "Read/Write Control"("FPGA VI Reference In"=w500, "hdt.int.p.readParams"=w501, "sicm.display"=w495) -> ("FPGA VI Reference Out"=w499:T6, "error out"=w498:errorcluster)  [unwired: 1 in]
        n220 = Add(x=w479, y=w486) -> (x+y=w487:dbl)
        n221 = property on="Graph" class="WFGraph (strict)"("Active Cursor"=u32 3, "Cursor.Cursor X"=w487) -> ()  [unwired: 2 in, 2 out]
      }
      frame "Reset.Background" {
        n222 = xnode "Read/Write Control"("FPGA VI Reference In"=w511, "error in"=w510) -> ("FPGA VI Reference Out"=w515:T6, "error out"=w514:errorcluster, "sicm.blc.p.params"=w509:T16)
        n223 = local read "Reset"() -> (w507:bool)
        n224 = Bundle By Name(cluster=w509, "blc.resetBackground"=w507) -> (w508:T16)
        n225 = xnode "Read/Write Control"("FPGA VI Reference In"=w515, "error in"=w514, "sicm.blc.p.params"=w508) -> ("FPGA VI Reference Out"=w513:T6, "error out"=w512:errorcluster)
      }
      frame "--------- IV-Curve ---------" {
      }
      frame "IV-Curve.Sweep" {
        # "max \nmin"
        n226 = xnode "Read/Write Control"("FPGA VI Reference In"=w532, "error in"=w533) -> ("FPGA VI Reference Out"=w531:T9, "error out"=w553:errorcluster, "aio.o.outputs"=w525:i16[])
        n227 = property on="Voltage\nRamp" class="Clust (strict)"() -> ("Value"=w527:cluster{"Min":dbl, "Max":dbl})  [unwired: 2 in, 2 out]
        n228 = Unbundle By Name(w527) -> ("Max"=w539:dbl, "Min"=w519:dbl)
        n229 = property on="Points" class="DigNum (strict)"() -> ("Value"=w526:i32)  [unwired: 2 in, 2 out]
        n230 = Subtract(x=w539, y=w519) -> (x-y=w540:dbl)
        n231 = Divide(x=w540, y=w526) -> (x/y=w541:dbl)
        n232 = for {
          N: w526 -> [_]
          tunnel: w541 -> [w585]
          tunnel: [w583] -> w521 mode=indexing
          i -> [w584]
          n233 = Multiply(x=w585, y=w584) -> (x*y=w583:dbl)
        }
        n234 = Initialize Array(0.0 ("element"), w526) -> (w549:dbl[])
        n235 = Add(x=w521, y=w519) -> (x+y=w520:dbl[])
        n236 = Multiply(x=w520, y=32678.0) -> (x*y=w543:dbl[])
        n237 = Add(x=w519, y=w520) -> (x+y=w534:dbl[])
        n238 = Divide(x=w543, y=w538) -> (x/y=w524:dbl[])
        n239 = Array Size(array=w524) -> (size(s)=w523:i32)
        n240 = for {
          tunnel: w524 -> [w575] mode=indexing
          tunnel: w531 -> [w572]
          tunnel: w553 -> [w571]
          shift-right: [w564] -> w550
          shift-left: w549 -> [w565]
          tunnel: u32 10 ("milliseconds to wait") -> [w563]
          tunnel: [w578] -> w529
          tunnel: [w579] -> w530
          tunnel: w523 -> [w559]
          tunnel: 100.0 -> [w556]
          i -> [w560]
          stop <- w562 continue-if-true
          n241 = xnode "Read/Write Control"("FPGA VI Reference In"=w572, "error in"=w571) -> ("FPGA VI Reference Out"=w574:T9, "error out"=w573:errorcluster, "aio.o.outputs"=w576:i16[])
          n242 = To Word Integer(number=w575) -> (16bit integer=w561:i16)
          n243 = Replace Array Subset(array=w576, new element=w561) -> (w577:i16[])  [unwired: 1 in]
          n244 = xnode "Read/Write Control"("FPGA VI Reference In"=w574, "error in"=w573, "aio.o.outputs"=w577) -> ("FPGA VI Reference Out"=w570:T9, "error out"=w569:errorcluster)
          n245 = Divide(x=w560, y=w559) -> (x/y=w557:dbl)
          n246 = Multiply(x=w557, y=w556) -> (x*y=w558:dbl)
          n247 = flat-sequence {
            tunnel: w570 -> [w582]
            tunnel: w569 -> [w581]
            tunnel: [w582] -> w568
            tunnel: [w581] -> w567
            tunnel: w563 -> [w580]
            frame #0 {
              n248 = Wait (ms)(milliseconds to wait=w580) -> ()  [unwired: 1 out]
            }
          }
          n249 = To Unsigned Byte Integer(number=w558) -> (unsigned 8bit integer=→"Progress":u8)
          n250 = xnode "Read/Write Control"("FPGA VI Reference In"=w568, "error in"=w567) -> ("FPGA VI Reference Out"=w579:T9, "error out"=w578:errorcluster, "aio.s.slowVertical"=w566:i16)
          n251 = property on="Ramp" class="Bool (strict)"() -> ("Value"=w562:bool)  [unwired: 2 in, 2 out]
          n252 = Insert Into Array(array=w565, index=w560, new element=w566) -> (w564:dbl[])
        }
        n253 = To Double Precision Float(number=w550) -> (double precision float=w547:dbl[])
        n254 = xnode "Read/Write Control"("FPGA VI Reference In"=w530, "error in"=w529, "aio.o.outputs"=w525) -> ("error out"=w528:errorcluster)  [unwired: 1 out]
        n255 = Scale By Power Of 2(n=i16 -15, x=w547) -> (x*2^n=w545:dbl[])
        n256 = Multiply(x=w545, y=10.0) -> (x*y=w552:dbl[])
        n257 = Bundle(w534, w552) -> (w537:cluster{dbl[], dbl[]})  [unwired: 1 in]
        "IV Curve" <- w537
        n258 = property on="Ramp" class="Bool (strict)"(error in=w528, "Value"=FALSE ("Ramp")) -> (error out=w536:errorcluster)  [unwired: 1 in, 1 out]
      }
      frame "IV-Curve.Condition" {
        w615 = 10.0  # Why
        w610 = 100.0  # Why
        # "R2"
        # "Z"
        # "XY"
        # "Inner Radius"
        # "Resistante"
        # "bias"
        # "cotan(Theta/2)"
        n259 = xnode "Read/Write Control"("FPGA VI Reference In"=w608, "error in"=w609) -> ("FPGA VI Reference Out"=w601:T6, "error out"=w602:errorcluster, "aio.s.slowVertical"=w605:i16)
        n260 = To Double Precision Float(number=w605) -> (double precision float=w597:dbl)
        n261 = Unbundle By Name("IVParameters") -> ("Gain"=w591:dbl, "Apex Angle"=w594:dbl, "Conductivity"=w593:dbl, "Solution"=w587:string)
        n262 = Divide(x=w597, y=32768.0) -> (x/y=w606:dbl)
        n263 = xnode "Read/Write Control"("FPGA VI Reference In"=w601, "error in"=w602) -> ("FPGA VI Reference Out"=w600:T6, "error out"=w599:errorcluster, "aio.o.outputs"=w603:i16[])
        n264 = Compound Arithmetic op=MULTIPLY(w588, w606, w591, 1000000000.0 ("y")) -> (w592:dbl)
        n265 = Decimal String To Number(string=w587) -> (number=w625:i32)  [unwired: 2 in, 1 out]
        n266 = Empty String/Path?(string/path=w587) -> (empty?=w586:bool)
        n267 = Select(t=w593, s=w586, f=w625) -> (s? t:f=w626:dbl)
        n268 = Index Array(array=w603) -> (element=w598:i16)  [unwired: 1 in]
        n269 = Divide(x=w626, y=w610) -> (x/y=w611:dbl)
        n270 = To Double Precision Float(number=w598) -> (double precision float=w596:dbl)
        n271 = Divide(x=w596, y=w592) -> (x/y=w589:dbl)
        "Resistance" <- w589
        n272 = Divide(x=w594, y=2.0) -> (x/y=w623:dbl)
        n273 = Cotangent(1:w623) -> (0:w622:dbl)
        n274 = Add(x=w615, y=w622) -> (x+y=w616:dbl)
        n275 = Divide(x=w616, y=w611) -> (x/y=w612:dbl)
        n276 = Divide(x=w612, y=3.141592653589793) -> (x/y=w613:dbl)
        n277 = Divide(x=w613, y=w589) -> (x/y=w619:dbl)
        "Inner radius" <- w619
        n278 = Multiply(x=w619, y=1.5) -> (x*y=→"XY":dbl)
        n279 = Divide(x=w619, y=5.0) -> (x/y=→"Z":dbl)
      }
      frame "Conductivity.Update" {
        # "Conductivity value\ndisable"
        n280 = Variant To Data(error in=w635, type="" ("NewVal"), Variant=w634) -> (data=w628:string, error out=w637:errorcluster)
        n281 = Empty String/Path?(string/path=w628) -> (empty?=w627:bool)
        n282 = case shown="False" w627 {
          tunnel: [w640 100.0] -> w632
          tunnel: w628 -> [w639 _]
          tunnel: [T11."Disabled and Grayed Out" ("Disabled") T11."Enabled" ("Disabled")] -> w631
          frame False {
            n283 = Decimal String To Number(string=w639) -> (number=w641:i32)  [unwired: 2 in, 1 out]
            n284 = To Double Precision Float(number=w641) -> (double precision float=w640:dbl)
          }
          frame True {
          }
        }
        n285 = property on="Conductivity" class="DigNum (strict)"(error in=w637, "Value"=w632, "DisabledEnum"=w631) -> (error out=w630:errorcluster)  [unwired: 1 in, 1 out]
      }
      frame "RealTime.Update" {
        n286 = Variant To Data(error in=w653, type=FALSE ("NewVal"), Variant=w652) -> (data=w645:bool, error out=w656:errorcluster)
        n287 = property on="IV Curve" class="XYGraph (strict)"(error in=w656, "Visible"=FALSE) -> (error out=w649:errorcluster)  [unwired: 1 in, 1 out]
        n288 = property on="RT Graph" class="WFChart (strict)"(error in=w649, "Visible"=w645) -> (error out=w644:errorcluster)  [unwired: 1 in, 1 out]
        n289 = Not(x=w645) -> (.not. x?=w646:bool)
        n290 = property on="Graph" class="WFGraph (strict)"(error in=w644, "Visible"=w646) -> (error out=w648:errorcluster)  [unwired: 1 in, 1 out]
        n291 = property on="Cursor" class="DigNum (strict)"(error in=w648, "Visible"=w646) -> (error out=w647:errorcluster)  [unwired: 1 in, 1 out]
      }
      frame "Plots.Show" {
        n292 = Variant To Data(error in=w673, type=refnum<vi> refnum ("CtlRef"), Variant=w670) -> (data=w669:refnum<vi>, error out=w668:errorcluster)
        n293 = property class="Bool (strict)"(reference=w669, error in=w668) -> (error out=w666:errorcluster, "Value"=w665:bool, "Label.Text"=w662:string)  [unwired: 1 out]
        n294 = control-ref of="Graph"() -> (w659:refnum<vi>)
        n295 = control-ref of="RT Graph"() -> (w657:refnum<vi>)
        n296 = property on="Graph" class="WFGraph (strict)"() -> ("Value"=w664:waveform(dbl)[])  [unwired: 2 in, 2 out]
        n297 = Array Size(array=w664) -> (size(s)=w660:i32)
        n298 = String Subset(string=w662, length (rest)=1 ("length (rest)")) -> (substring=w661:string)  [unwired: 1 in]
        n299 = for {
          N: w660 -> [_]
          tunnel: w661 -> [w680]
          tunnel: w659 -> [w678]
          tunnel: [w681] -> w674
          tunnel: w657 -> [w676]
          i -> [w675]
          stop <- w679 stop-if-true
          n300 = property class="WFGraph (strict)"(reference=w678, "Active Plot"=w675) -> (error out=w681:errorcluster, "Plot.Plot Name"=w677:string)  [unwired: 1 in, 1 out]
          n301 = property class="WFChart (strict)" props=["Active Plot", "Plot", "Plot Name"](reference=w676, "Active Plot"=w675) -> ()  [unwired: 1 in, 3 out]
          n302 = Equal?(x=w680, y=w677) -> (x = y?=w679:bool)
        }
        n303 = property on="RT Graph" class="WFChart (strict)"(error in=w674, "Plot.Visible?"=w665) -> (error out=w658:errorcluster)  [unwired: 1 in, 1 out]
        n304 = property on="Graph" class="WFGraph (strict)"(error in=w658, "Plot.Visible?"=w665) -> ()  [unwired: 1 in, 2 out]
      }
      frame "Thumbnail.TabChange" {
        n305 = Variant To Data(error in=w697, type=0, Variant=w695) -> (data=w692:i32, error out=w696:errorcluster)
        n306 = property on="SICM" class="TabCtl (strict)"(error in=w696) -> (error out=w703:errorcluster, "Pages"=w693:refnum<vi>[])  [unwired: 1 in, 1 out]
        n307 = Index Array(array=w693, index=w692) -> (element=w691:refnum<vi>)
        n308 = property class="Page"(reference=w691, error in=w703) -> (error out=w698:errorcluster, "PageLabel"=w700:string)  [unwired: 1 out]
        n309 = Equal?(x=w700, y="IV Curve") -> (x = y?=w688:bool)
        n310 = case shown="False" w688 {
          selector: w688 -> [w704 w710]
          tunnel: [w709 w711] -> w690
          tunnel: [w706 w711] -> w689
          tunnel: [TRUE w711] -> w686
          tunnel: [w705 w712] -> w685
          tunnel: [w705 w712] -> w684
          tunnel: [w705 w711] -> w683
          tunnel: [w704 w710] -> w682
          frame False {
            n311 = Not(x=w704) -> (.not. x?=w705:bool)
            n312 = property on="Real Time" class="Bool (strict)"("Visible"=w705) -> (error out=w707:errorcluster)  [unwired: 2 in, 1 out]
            n313 = property on="Real Time" class="Bool (strict)"(error in=w707) -> ("Value"=w706:bool)  [unwired: 1 in, 2 out]
            n314 = Not(x=w706) -> (.not. x?=w709:bool)
          }
          frame True {
            w711 = FALSE
            n315 = Not(x=w710) -> (.not. x?=w712:bool)
          }
        }
        n316 = property on="IV Curve" class="XYGraph (strict)"(error in=w698, "Visible"=w688) -> (error out=w687:errorcluster)  [unwired: 1 in, 1 out]
        n317 = property on="Real Time" class="Bool (strict)"("Visible"=w686) -> ()  [unwired: 2 in, 2 out]
        n318 = property on="RT Graph" class="WFChart (strict)"("Visible"=w689) -> ()  [unwired: 2 in, 2 out]
        n319 = property on="Graph" class="WFGraph (strict)"("Visible"=w690) -> ()  [unwired: 2 in, 2 out]
        n320 = property on="Plots" class="Clust (strict)"("Visible"=w684) -> ()  [unwired: 2 in, 2 out]
        n321 = property on="Baseline" class="DigNum (strict)"("Visible"=w685) -> ()  [unwired: 2 in, 2 out]
        n322 = property on="Update" class="DigNum (strict)"("Visible"=w683) -> ()  [unwired: 2 in, 2 out]
        n323 = property on="Progress" class="Slide (strict)"("Visible"=w682) -> ()  [unwired: 2 in, 2 out]
        n324 = property on="Height" class="DigNum (strict)"("Visible"=w685) -> ()  [unwired: 2 in, 2 out]
        n325 = property on="Current" class="DigNum (strict)"("Visible"=w685) -> ()  [unwired: 2 in, 2 out]
        n326 = property on="Trig Height" class="DigNum (strict)"("Visible"=w685) -> ()  [unwired: 2 in, 2 out]
      }
      frame "ZController.IOFrequency" {
        n327 = call "Enqueue Message.vi"("error in"=w718, "Data"="Adaptive", "Message"="Adaptive.Update", "Queue"=w726) -> ("error out"=w717:errorcluster, "Queue dup."=w725:refnum<queue>)  [unwired: 6 in]
        n328 = call "Enqueue Message.vi"("error in"=w717, "Message"="Retract.Update", "Queue"=w725) -> ("error out"=w713:errorcluster, "Queue dup."=w724:refnum<queue>)  [unwired: 7 in]
        n329 = property on="Window" class="Clust (strict)"(error in=w713) -> (error out=w727:errorcluster, "Value"=w714:cluster{"Window":dbl})  [unwired: 1 in, 1 out]
        n330 = call "Enqueue Message.vi"("error in"=w727, "Data"=w714, "Message"="Length.Update", "Queue"=w724) -> ("error out"=w716:errorcluster)  [unwired: 6 in, 1 out]
      }
      frame "Exit" {
        w730 = u8 0 items=["ORT", "SICM"] ("hdt.mainOutStreamSelect")
        w736 = u8 0 items=["PID/ORT", "SICM"] ("hdt.mainOutStreamSelect")
        n331 = Release Queue(queue=w742, error in (no error)=w741) -> (error out=w737:errorcluster)  [unwired: 1 in, 2 out]
        n332 = xnode "Read/Write Control"("FPGA VI Reference In"=w739, "error in"=w737, "flt.bypassPI"=FALSE, "hdt.mainOutStreamSelect"=w736, "hdt.int.p.memWriteSource"=w730, "flt.bypassPI"=FALSE) -> ("FPGA VI Reference Out"=w738:T6, "error out"=w733:errorcluster)
        n333 = call "Fire User Event - Stop.vi"("Événement utilisateur - Arrêt"=w735) -> ("sortie d'erreur"=w734:errorcluster)  [unwired: 10 in]
        n334 = Merge Errors(w734, w733) -> (w732:errorcluster)
      }
      frame Default {
        n335 = Format Into String(format string="The message\"%s\" received in the gestion loop is not valid" ("Texte de message d'erreur inconnu"), w748) -> (resulting string=w745:string)  [unwired: 2 in, 1 out]
        n336 = call <vilib>:"Error Cluster From Error Code.vi"("error message (\"\")"=w745, "error code (0)"=1 ("code d'erreur (0)")) -> ("error out"=w746:errorcluster)  [unwired: 7 in]
      }
    }
  }
  n337 = while {
    shift-right: [w756] -> w43
    shift-left: w63 -> [w759]
    tunnel: w49 -> [w758]
    tunnel: w42 -> [w755]
    tunnel: w14 -> [w754]
    tunnel: w11 -> [w753]
    shift-right: [w751] -> _
    shift-left: w8 -> [w750]
    stop <- w757 stop-if-true
    n338 = event shown="[0] Timeout" {
      selector: w758 -> [_ _ _]
      dyn-events: _ -> [_ _ _]
      timeout: "Update" -> [w760 _ _]
      tunnel: w759 -> [w780 w847 w849]
      tunnel: [_ TRUE _] -> w757
      tunnel: [w782 w847 w849] -> w756
      tunnel: w755 -> [w772 _ _]
      tunnel: w754 -> [w765 _ _]
      tunnel: w753 -> [w768 _ _]
      tunnel: [w763 w846 w853] -> w751
      tunnel: w750 -> [w762 w846 w853]
      event Timeout {
        # "Current\nBaseline\nHeight\nTrigger"
        n339 = event-data() -> ()  [unwired: 1 in, 1 out]
        n340 = local read "Real Time"() -> (w761:bool)
        n341 = xnode "Read/Write Control"("FPGA VI Reference In"=w780) -> ("aio.s.slowVertical"=w776:i16, "sicm.s.baseline"=w781:T20, "sicm.o.height"=w774:fxp<+/-,28,2>, "sicm-hdt.t.triggerHeight"=w779:fxp<+/-,22,4>)  [unwired: 1 in, 2 out]
        n342 = Unbundle By Name(w781) -> ("carryOut"=w773:fxp<+/-,22,2>)
        n343 = To Double Precision Float(number=w776) -> (double precision float=w778:dbl)
        n344 = To Double Precision Float(number=w773) -> (double precision float=w764:dbl)
        n345 = To Double Precision Float(number=w774) -> (double precision float=w771:dbl)
        n346 = To Double Precision Float(number=w779) -> (double precision float=w766:dbl)
        n347 = case shown="False" w761 {
          tunnel: [w797 w839] -> w782
          tunnel: w780 -> [w790 w839]
          tunnel: w766 -> [w789 _]
          tunnel: w764 -> [w785 _]
          tunnel: w765 -> [w788 _]
          tunnel: [w787 w838] -> w763
          tunnel: w762 -> [w786 w838]
          tunnel: w760 -> [w784 _]
          frame False {
            n348 = xnode "Invoke Method"("FPGA VI Reference In"=w790, "IRQ Number(s)"=5, "Timeout (ms)"=200) -> ("FPGA VI Reference Out"=w795:T6, "error out"=w794:errorcluster, "Timed Out"=w791:bool)  [unwired: 1 in, 1 out]
            n349 = Not(x=w791) -> (.not. x?=w796:bool)
            n350 = case shown="True" w796 {
              tunnel: w794 -> [w806 w821]
              tunnel: w795 -> [w807 w812]
              tunnel: [w805 w822] -> w797
              tunnel: [w804 w823] -> _
              tunnel: w789 -> [_ w815]
              tunnel: w788 -> [_ w818]
              tunnel: [w798 w816] -> w787
              tunnel: w786 -> [w798 w834]
              tunnel: w785 -> [_ w814]
              tunnel: w784 -> [_ w813]
              frame False {
                # "invert the channel at every read of the memory"
                n351 = xnode "Read/Write Control"("FPGA VI Reference In"=w807, "error in"=w806) -> ("FPGA VI Reference Out"=w801:T6, "error out"=w800:errorcluster, "hdt.int.p.readParams"=w799:T17)
                n352 = Bundle By Name(cluster=w799, "hdt.int.p.startTransfer"=TRUE) -> (w803:T17)
                n353 = xnode "Read/Write Control"("FPGA VI Reference In"=w801, "error in"=w800, "hdt.int.p.readParams"=w803) -> ("FPGA VI Reference Out"=w805:T6, "error out"=w804:errorcluster)
              }
              frame True {
                n354 = xnode "Read/Write Control"("FPGA VI Reference In"=w812) -> ("sicm.display.sicm.p.memorywWriteDec"=w811:u16)  [unwired: 1 in, 2 out]
                n355 = flat-sequence {
                  tunnel: w821 -> [w836]
                  tunnel: [w836] -> w827
                  tunnel: [w835] -> w826
                  tunnel: w812 -> [w835]
                  frame #0 {
                    n356 = Wait (ms)(milliseconds to wait=u32 10) -> ()  [unwired: 1 out]
                  }
                }
                n357 = xnode "Invoke Method"("FPGA VI Reference In"=w826, "error in"=w827, "Number of Elements"=u32 0, "Timeout (ms)"=20) -> ("FPGA VI Reference Out"=w829:T6, "error out"=w828:errorcluster, "Elements Remaining"=w832:u32)  [unwired: 1 out]
                n358 = call "FGVSamplingRates.vi"("Enum"=Enum."Read") -> ("samplingRatesOut"=w819:T15)  [unwired: 9 in, 1 out]
                n359 = xnode "Invoke Method"("FPGA VI Reference In"=w829, "error in"=w828, "Number of Elements"=w832, "Timeout (ms)"=w813) -> ("FPGA VI Reference Out"=w824:T6, "error out"=w833:errorcluster, "Data"=w817:i16[])  [unwired: 1 out]
                n360 = Unbundle By Name(w819) -> ("feedbackHz"=w810:u32)
                n361 = Bundle(cluster=T19 {"feedbackHz"=0, "sicm.display.sicm.p.memorywWriteDec"=0}, "feedbackHz"=w810, "sicm.display.sicm.p.memorywWriteDec"=w811) -> (w809:T19)
                n362 = xnode "Invoke Method"("FPGA VI Reference In"=w824, "error in"=w833, "IRQ Number(s)"=5) -> ("FPGA VI Reference Out"=w822:T6, "error out"=w823:errorcluster)
                n363 = call "SICMDisplayGraph.vi"("Baseline"=w814, "Data"=w817, "TriggerHeight"=w815, "TimeRes"=w809, "voltageRange"=w818, "ArrayToReplace"=w834) -> ("Graph"=w816:waveform(dbl)[])  [unwired: 5 in]
                "Graph" <- w816
              }
            }
          }
          frame True {
          }
        }
        n364 = Multiply(x=w771, y=w768) -> (x*y=w770:dbl)
        "Height" <- w770
        n365 = Multiply(x=w766, y=w768) -> (x*y=w769:dbl)
        "Trig Height" <- w769
        n366 = Multiply(x=w765, y=w764) -> (x*y=w783:dbl)
        "Baseline" <- w783
        n367 = Scale By Power Of 2(n=i16 -15, x=w778) -> (x*2^n=w775:dbl)
        n368 = Multiply(x=w772, y=w775) -> (x*y=w767:dbl)
        "Current" <- w767
        n369 = case shown="True" w761 {
          tunnel: w783 -> [_ w845]
          tunnel: w769 -> [_ w844]
          tunnel: w767 -> [_ w843]
          tunnel: w770 -> [_ w842]
          frame False {
          }
          frame True {
            n370 = Build Array(w845, w843, w842, w844) -> (w841:dbl[])
            n371 = Build Array(w841) -> (→"RT Graph":dbl[][])
          }
        }
      }
      event User Event {
        n372 = event-data() -> ()  [unwired: 1 in, 4 out]
      }
      event "Update": Value Change {
        n373 = event-data() -> ("NewVal"=w850:i32)  [unwired: 1 in]
        n374 = Compound Arithmetic op=MULTIPLY(0.001, w850) -> (w852:dbl)
        n375 = property on="RT Graph" class="WFChart (strict)"("XScale.Multiplier"=w852) -> ()  [unwired: 2 in, 2 out]
      }
    }
  }
  n376 = Merge Errors(w56, w57) -> (w48:errorcluster)
  n377 = call "Destroy User Event - Stop.vi"("entrée d'erreur (pas d'erreur)"=w48, "Événement utilisateur - Arrêt"=w46) -> ("sortie d'erreur"=w47:errorcluster)  [unwired: 9 in]
  n378 = flat-sequence {
    tunnel: w47 -> [w854]
    frame #0 {
      n379 = call <vilib>:"Simple Error Handler.vi"("error in (no error)"=w854) -> ()  [unwired: 4 in, 5 out]
    }
    frame #1 {
      n380 = Request Deallocation(TRUE ("flag")) -> ()
    }
  }
  n381 = xnode "Invoke Method"("FPGA VI Reference In"=w43) -> ()  [unwired: 1 in, 2 out]
